vi "ADC_ADMode.vi"(7 "DeviceIndex":u32, 8 "error in (no error)":errorcluster) -> (0 "error out":errorcluster)   [LabVIEW 2012]
doc: "unsigned long ADC_ADMode(\nunsigned long DeviceIndex - number from 0-31 indicating on which device you wish to set\noverall A/D parameters\nunsigned char TriggerMode - byte indicating which A/D trigger source to use, see the manual for\ndetails. Also sets the clock source for counter 0\nunsigned char CalMode - byte indicating which A/D source to use - 00 hex for actual inputs, 01\nhex for calibration ground reference, 02 hex for calibration high reference. Other values cause the\ncall to fail, returning \"ERROR_INVALID_PARAMETER\"(equal to 87 decimal).\n)\nOn the USB-AI12-16E, calibration references are not included, and calibration modes of 01 and\n02 will be treated as 00. This function is still used to set the trigger mode."
uses:
  Controls/Calibration Mode (ADMode).ctl
  Windows/System32/AIOUSB.dll
panel:
  in  "CalMode":T1
  in  "TriggerMode":u8
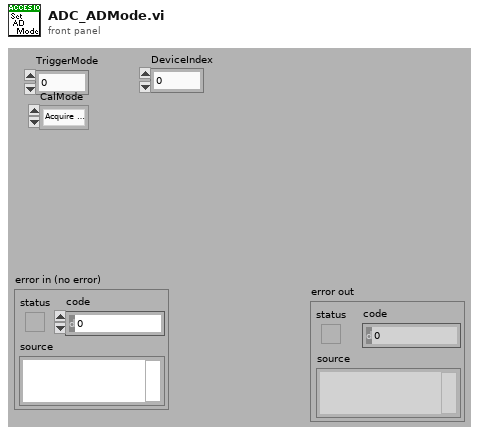
[diagram p1: front panel]
types:
  T1 = typedef "Calibration Mode (ADMode).ctl" = enum8{"Acquire Data", "Acquire Ground", "Do not use", "Aquire Cal. Ref."}
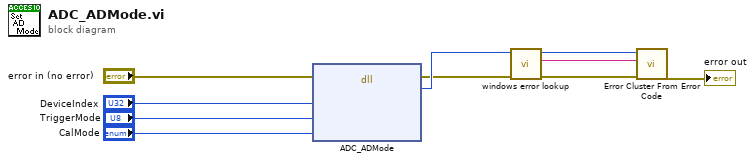
[diagram p0: block diagram]
diagram:
  n1 = dll-call lib="C:/Windows/System32/AIOUSB.dll" fn="ADC_ADMode"(error in="error in (no error)", "DeviceIndex"="DeviceIndex", "TriggerMode"="TriggerMode", "CalMode"="CalMode") -> (error out=w4:errorcluster, "return type"=w5:u32)  [unwired: 5 in, 1 out]
  n2 = call "windows error lookup.vi"("error in (no error)"=w4, "Error Code"=w5) -> ("error out"=w3:errorcluster, "error message (\"\")"=w6:string)  [unwired: 8 in]
  n3 = call <vilib>:"Error Cluster From Error Code.vi"("error in (no error)"=w3, "error message (\"\")"=w6, "error code (0)"=w5) -> ("error out"=→"error out":errorcluster)  [unwired: 6 in]
